vi "Input Section.vi"(8 "error in (no error)":errorcluster, 11 "Node Ptr":T1 format="%.0x") -> (0 "error out":errorcluster)   [LabVIEW 2021, in "DAQ Analog InOut System Explorer.lvlib"]
uses:
  DAQ Analog InOut System Explorer.lvlib
  <vilib>/NI VeriStand/Custom Device API/Custom Device Item Ref.ctl
  Shared/Constants.vi
  <vilib>/NI VeriStand/Custom Device API/Get Item Property (Double).vi
  <vilib>/NI VeriStand/Custom Device API/Set Item Property (Double).vi
  <vilib>/NI VeriStand/Custom Device API/Custom Device API.lvlib
  Shared/DAQ Analog InOut Shared.lvlib
panel:
  in  "AI Sample Rate":dbl
  in  "General Header":cluster{"Section Name":string}={"Section Name"="General Page Settings"}
  in  "Description":string
  in  "Name":string
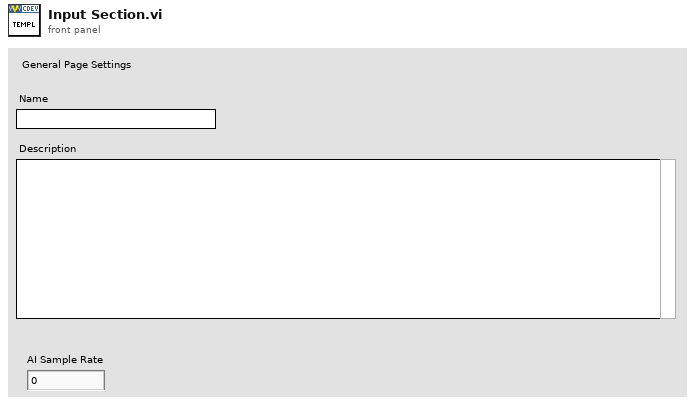
[diagram p1: front panel]
types:
  T1 = typedef "Custom Device API.lvlib/Custom Device Item Ref.ctl" = u64
  T2 = typedef "Custom Device API.lvlib/Custom Device Item Info.ctl" = cluster{"Name":string, "Is Channel":bool, "GUID":string, "Is Waveform":bool}
  T3 = typedef "Custom Device API.lvlib/Custom Device Commands.ctl" = enum16{"Default", "Item renamed", "Shutdown", "Dynamic button pressed"}
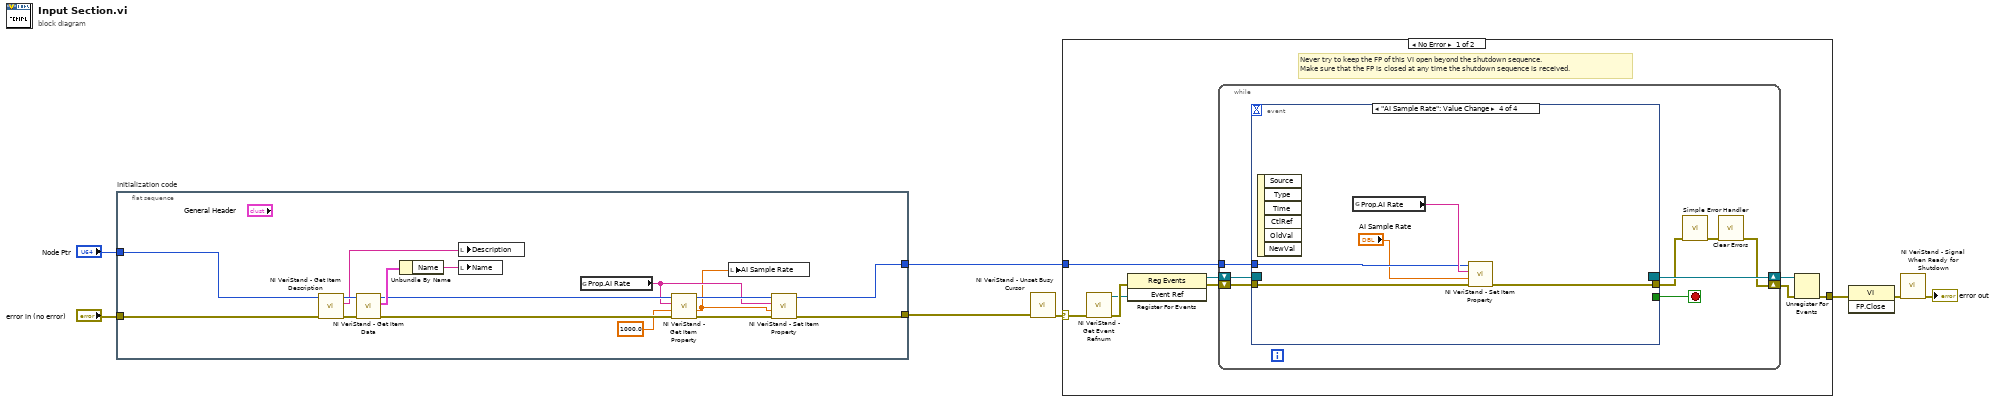
[diagram p0: block diagram]
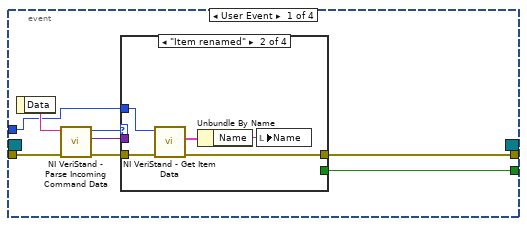
[diagram p2: hidden frame]
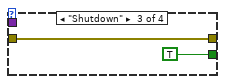
[diagram p4: hidden frame]
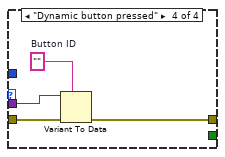
[diagram p5: hidden frame]
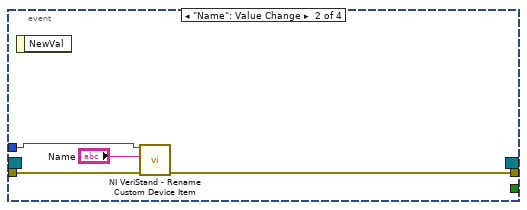
[diagram p6: hidden frame]
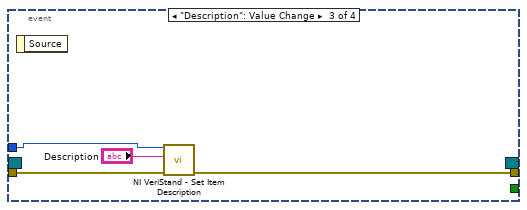
[diagram p7: hidden frame]
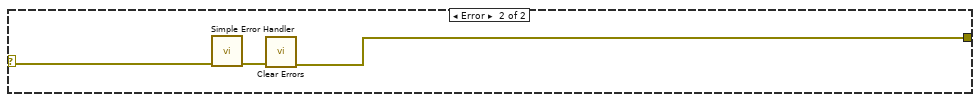
[diagram p8: hidden frame]
diagram:
  n1 = flat-sequence "Initialization code" {
    tunnel: "error in (no error)" -> [w18]
    tunnel: "Node Ptr" -> [w22]
    tunnel: [w9] -> w2
    tunnel: [w10] -> w1
    frame #0 {
      n2 = call <vilib>:"NI VeriStand - Get Item Description.vi"("error in (no error)"=w18, "Item Ref in"=w22) -> ("error out"=w23:errorcluster, "Description"=w20:string, "Item Ref out"=w24:T1)  [unwired: 7 out]
      n3 = call <vilib>:"NI VeriStand - Get Item Data.vi"("error in (no error)"=w23, "Item Ref in"=w24) -> ("error out"=w16:errorcluster, "Item Info"=w19:T2, "Item Ref out"=w17:T1)  [unwired: 7 out]
      n4 = Unbundle By Name(w19) -> ("Name"=w21:string)
      n5 = local write "Description"(w20) -> ()
      n6 = local write "Name"(w21) -> ()
      n7 = global read "Constants.vi" "Prop.AI Rate"() -> (w12:string)
      n8 = call-poly <vilib>:"NI VeriStand - Get Item Property.vi"("error in (no error)"=w16, "Default Value"=1000.0 ("Value"), "Property Name"=w12, "Item Ref in"=w17) -> ("error out"=w13:errorcluster, "Value"=w11:dbl, "Item Ref out"=w14:T1)  [unwired: 4 in, 1 out]
      n9 = local write "AI Sample Rate"(w11) -> ()
      n10 = call-poly <vilib>:"NI VeriStand - Set Item Property.vi"("error in (no error)"=w13, "Value"=w11, "Property Name"=w12, "Item Ref in"=w14) -> ("error out"=w9:errorcluster, "Item Ref out"=w10:T1)  [unwired: 5 in, 1 out]
    }
  }
  n11 = call <vilib>:"NI VeriStand - Unset Busy Cursor.vi"("error in (no error)"=w2) -> ("error out"=w4:errorcluster)  [unwired: 10 out]
  n12 = case shown="No Error" w4 {
    selector: w4 -> [w26 w77]
    tunnel: [w30 w75] -> w8
    tunnel: w1 -> [w25 _]
    frame No Error {
      # "Never try to keep the FP of this VI open beyond the shutdown sequence.\nMake sure that the FP is closed at any time the shutdown sequence is received."
      n13 = call <vilib>:"NI VeriStand - Get Event Refnum.vi"("error in (no error)"=w26) -> ("error out"=w33:errorcluster, "Event Ref"=w29:refnum<user-event>)  [unwired: 9 out]
      n14 = register-events(error in=w33, w29) -> (reference out=w27:refnum<event-registration>, error out=w28:errorcluster)  [unwired: 1 in]
      n15 = while {
        shift-right: [w35] -> w31
        shift-left: w28 -> [w40]
        shift-right: [w41] -> w32
        shift-left: w27 -> [w39]
        tunnel: w25 -> [w34]
        stop <- w38 stop-if-true
        n16 = event shown="[3] \"AI Sample Rate\": Value Change" {
          selector: w39 -> [_ _ _ _]
          dyn-events: [_ _ _ _] -> w41
          timeout: _ -> [_ _ _ _]
          tunnel: w40 -> [w49 w65 w69 w72]
          tunnel: [w45 _ _ _] -> w38
          tunnel: [w44 w64 w68 w70] -> w37
          tunnel: w34 -> [w42 w62 w66 w73]
          event User Event {
            n17 = event-data() -> ("Data"=w48:string)  [unwired: 1 out]
            n18 = call <vilib>:"NI VeriStand - Parse Incoming Command Data.vi"("error in (no error)"=w49, "Incoming data"=w48) -> ("error out"=w47:errorcluster, "Outgoing data"=w43:variant, "Action"=w46:T3)  [unwired: 7 out]
            n19 = case shown="\"Item renamed\"" w46 {
              tunnel: w47 -> [w50 w55 w56 w61]
              tunnel: [_ _ TRUE _] -> w45
              tunnel: [w50 w53 w56 w58] -> w44
              tunnel: w43 -> [_ _ _ w60]
              tunnel: w42 -> [_ w51 _ _]
              frame "Default", Default {
              }
              frame "Item renamed" {
                n20 = call <vilib>:"NI VeriStand - Get Item Data.vi"("error in (no error)"=w55, "Item Ref in"=w51) -> ("error out"=w53:errorcluster, "Item Info"=w54:T2)  [unwired: 8 out]
                n21 = Unbundle By Name(w54) -> ("Name"=w52:string)
                n22 = local write "Name"(w52) -> ()
              }
              frame "Shutdown" {
              }
              frame "Dynamic button pressed" {
                w59 = ""  # Button ID
                n23 = Variant To Data(error in=w61, type=w59, Variant=w60) -> (error out=w58:errorcluster)  [unwired: 1 out]
              }
            }
          }
          event "Name": Value Change {
            n24 = event-data() -> ()  [unwired: 2 out]
            n25 = call <vilib>:"NI VeriStand - Rename Custom Device Item.vi"("error in (no error)"=w65, "New Name"="Name", "Item Ref in"=w62) -> ("error out"=w64:errorcluster)  [unwired: 1 in, 7 out]
          }
          event "Description": Value Change {
            n26 = event-data() -> ()  [unwired: 2 out]
            n27 = call <vilib>:"NI VeriStand - Set Item Description.vi"("error in (no error)"=w69, "Description"="Description", "Item Ref in"=w66) -> ("error out"=w68:errorcluster)  [unwired: 8 out]
          }
          event "AI Sample Rate": Value Change {
            n28 = event-data() -> ()  [unwired: 7 out]
            n29 = global read "Constants.vi" "Prop.AI Rate"() -> (w74:string)
            n30 = call-poly <vilib>:"NI VeriStand - Set Item Property.vi"("error in (no error)"=w72, "Value"="AI Sample Rate", "Property Name"=w74, "Item Ref in"=w73) -> ("error out"=w70:errorcluster)  [unwired: 5 in, 2 out]
          }
        }
        n31 = call <vilib>:"Simple Error Handler.vi"("error in (no error)"=w37) -> ("error out"=w36:errorcluster)  [unwired: 1 in, 7 out]
        n32 = call <vilib>:"Clear Errors.vi"("error in (no error)"=w36) -> ("error out"=w35:errorcluster)  [unwired: 1 in, 5 out]
      }
      n33 = Unregister For Events(event registration refnum=w32, error in=w31) -> (error out=w30:errorcluster)
    }
    frame Error {
      n34 = call <vilib>:"Simple Error Handler.vi"("error in (no error)"=w77) -> ("error out"=w76:errorcluster)  [unwired: 1 in, 7 out]
      n35 = call <vilib>:"Clear Errors.vi"("error in (no error)"=w76) -> ("error out"=w75:errorcluster)  [unwired: 1 in, 5 out]
    }
  }
  n36 = invoke class="VI" method="FP.Close"(error in=w8) -> (error out=w7:errorcluster)  [unwired: 2 in, 2 out]
  n37 = call <vilib>:"NI VeriStand - Signal When Ready for Shutdown.vi"("error in (no error)"=w7) -> ("error out"=→"error out":errorcluster)  [unwired: 10 out]
